vi "Lockin.Engine.vi"(8 "error in (no error)":errorcluster, 11 "DSP in":refnum<class "DSP.lvclass">) -> (0 "error out":errorcluster, 1 "Downsampled Waveforms":T1, 2 "Results":T2 {"Results (Dictionary)"."value" format="%#_6p"}, 3 "DSP out":refnum<class "DSP.lvclass">, 5 "Continue DSP?":bool)   [LabVIEW 2019, in "DSP.lvclass"]
uses:
  DSP.lvclass
  Typedefs/Results--Cluster.ctl
  Typedefs/Results Dictionary--Cluster.ctl
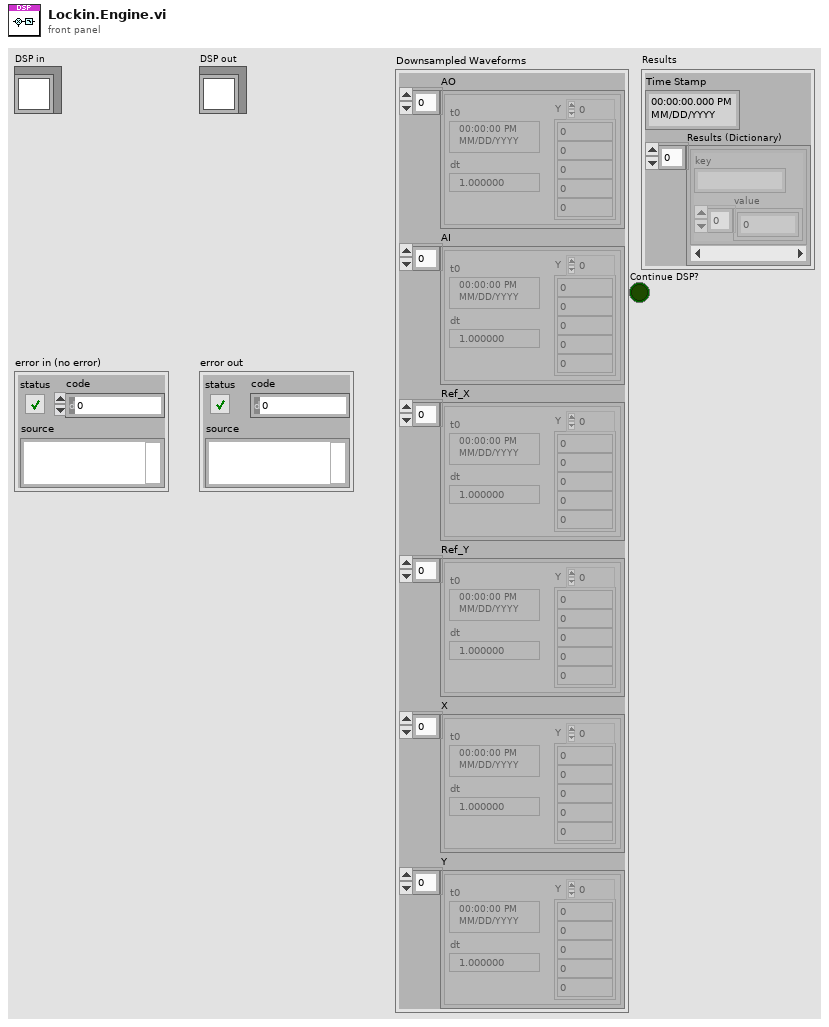
[diagram p1: front panel]
types:
  T1 = cluster{"AO":waveform(dbl)[], "AI":waveform(dbl)[], "Ref_X":waveform(dbl)[], "Ref_Y":waveform(dbl)[], "X":waveform(dbl)[], "Y":waveform(dbl)[]}
  T2 = typedef "DSP.lvclass/Results--Cluster.ctl" = cluster{"Time Stamp":timestamp, "Results (Dictionary)":T3[]}
  T3 = typedef "DSP.lvclass/Results Dictionary--Cluster.ctl" = cluster{"key":string, "value":dbl[]}
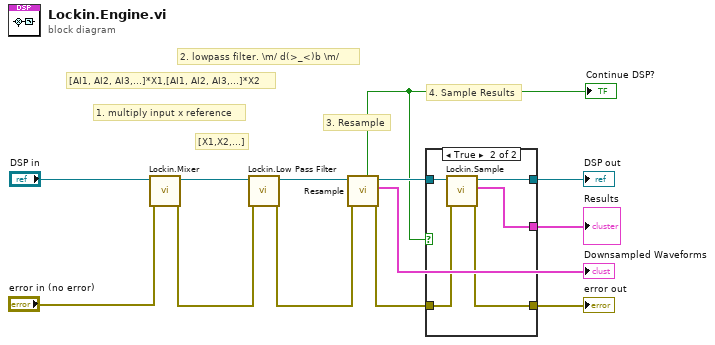
[diagram p0: block diagram]
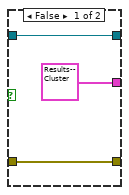
[diagram p2: hidden frame]
diagram:
  # "4. Sample Results"
  # "3. Resample"
  # "[X1,X2,...]"
  # "1. multiply input x reference"
  # "2. lowpass filter. \\m/ d(>_<)b \\m/"
  # "[AI1, AI2, AI3,...]*X1,[AI1, AI2, AI3,...]*X2"
  n1 = call "Lockin.Mixer.vi"("error in (no error)"="error in (no error)", "DSP in"="DSP in") -> ("error out"=w6:errorcluster, "DSP out"=w5:refnum<class "DSP.lvclass">)  [unwired: 8 in]
  n2 = call "Lockin.Low Pass Filter.vi"("error in (no error)"=w6, "DSP in"=w5) -> ("error out"=w8:errorcluster, "DSP out"=w7:refnum<class "DSP.lvclass">)  [unwired: 8 in]
  n3 = call "Resample.vi"("error in (no error)"=w8, "DSP in"=w7) -> ("error out"=w11:errorcluster, "Waveforms"=→"Downsampled Waveforms":T1, "DSP out"=w9:refnum<class "DSP.lvclass">, "Continue DSP?"=w1:bool)  [unwired: 6 in]
  "Continue DSP?" <- w1
  n4 = case shown="True" w1 {
    tunnel: [w14 w21] -> w13
    tunnel: [w16 w20] -> w12
    tunnel: w11 -> [w16 w19]
    tunnel: [T2 {"Time Stamp"=timestamp(0 s since 1904-01-01), "Results (Dictionary)"=[]} ("Results") w18] -> w10
    tunnel: w9 -> [w14 w17]
    frame False {
    }
    frame True {
      n5 = call "Lockin.Sample.vi"("error in (no error)"=w19, "DSP in"=w17) -> ("error out"=w20:errorcluster, "Results"=w18:T2, "DSP in"=w21:refnum<class "DSP.lvclass">)  [unwired: 7 in]
    }
  }
  "DSP out" <- w13
  "error out" <- w12
  "Results" <- w10
